vi "avitolcm.vi"() -> ()   [LabVIEW 2015]
uses:
  G_LCM.vi
panel:
  out "error out":errorcluster
  in  "Image 2":T1(plugin-control)
  in  "port":u16=7667
  in  "time-to-live":u16
  out "Image":T1(plugin-control)
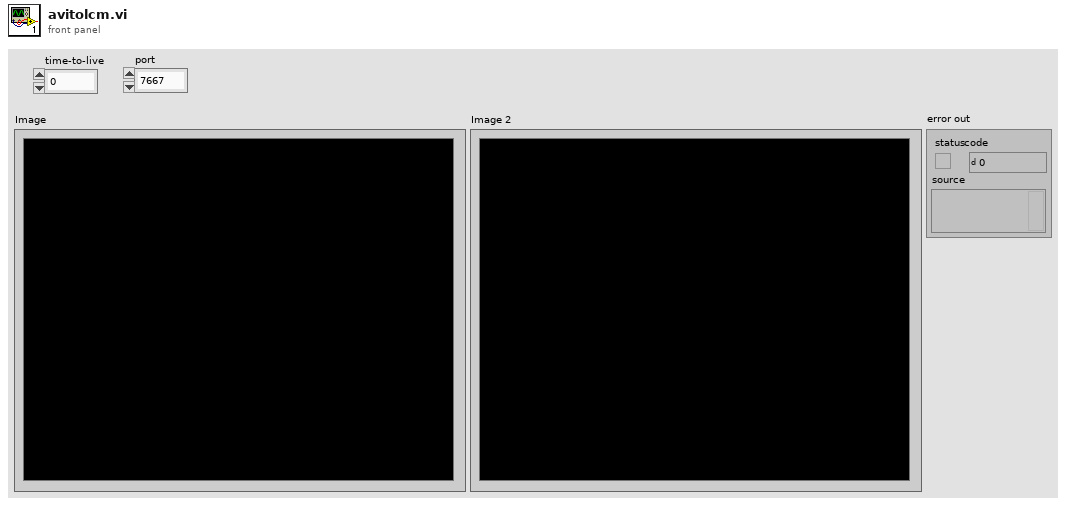
[diagram p1: front panel]
types:
  T1 = typedef "IMAQ Image.ctl" = refnum<image>
  T2 = cluster{"connection ID":refnum<k16>, "net address":u32, "port":u16}
  T3 = cluster{"hash":i64, "sys time":i64, "width":i32, "height":i32, "size":i32, "data":i32[]}
  T4 = typedef "IMAQ AVI2 Refnum.ctl" = refnum<k20>
  T5 = typedef "Image Type" = u32
  T6 = cluster{"Width":u32, "Height":u32, "Frames Per Second":u32, "Codec":string, "Has Data":bool}
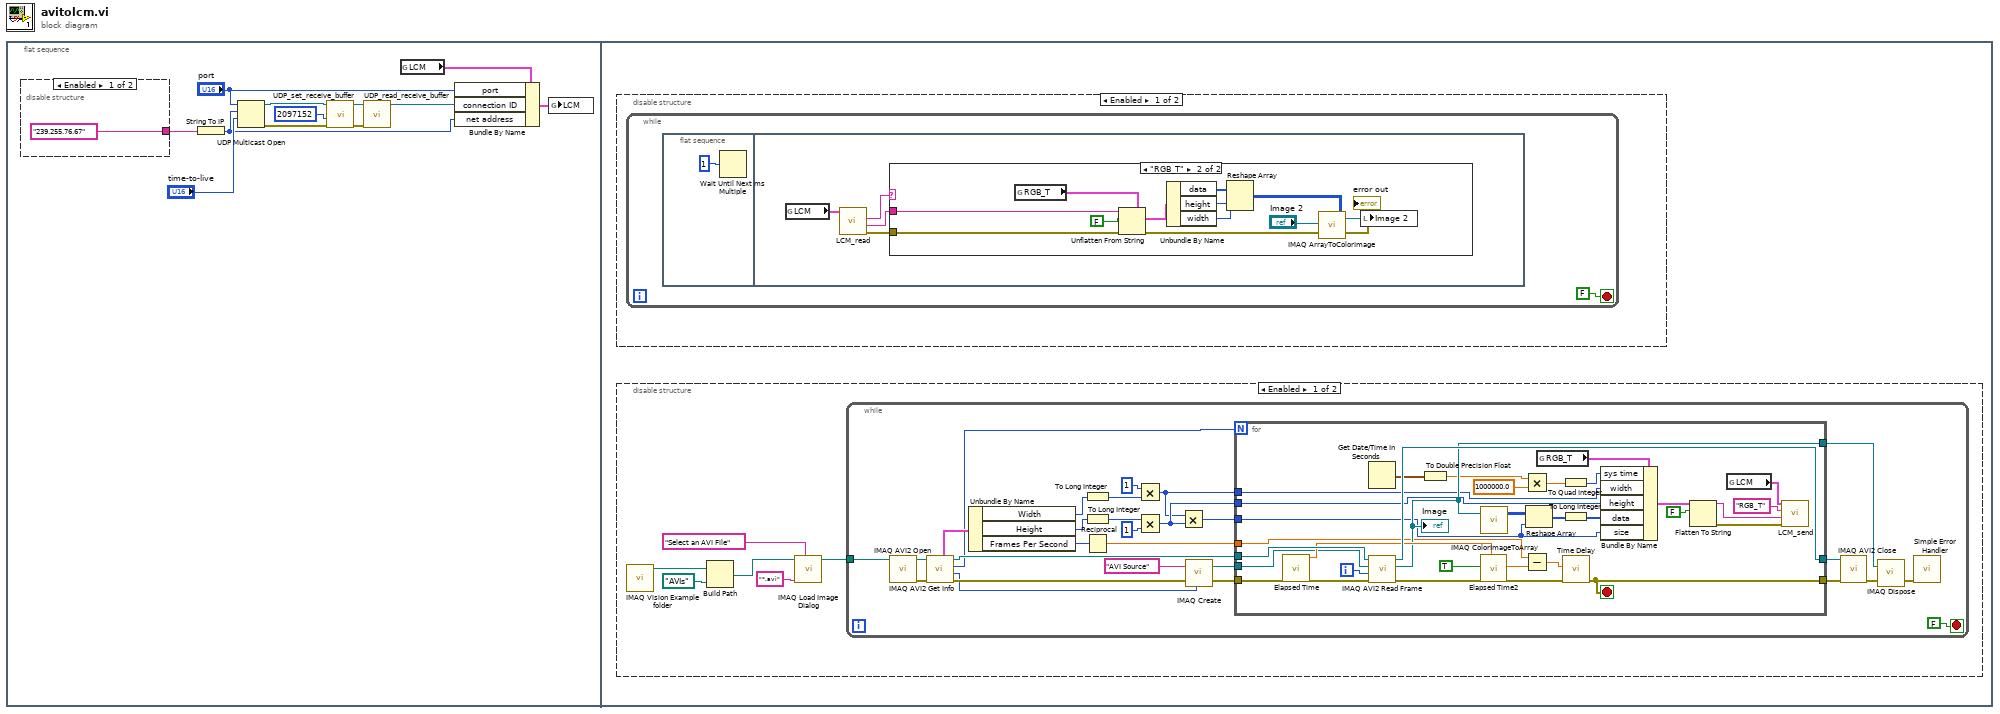
[diagram p0: block diagram]
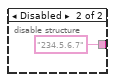
[diagram p2: hidden frame]
diagram:
  n1 = flat-sequence {
    frame #0 {
      n2 = disable-structure shown="Enabled" {
        disable-tunnel: ["239.255.76.67" ("Multicast Address") "234.5.6.7" ("Multicast Address")] -> w12
        frame Enabled {
        }
        frame Disabled {
        }
      }
      n3 = String To IP(1:w12) -> (0:w8:u32)
      n4 = UDP Multicast Open(9:"time-to-live", 10:w8, 11:"port") -> (0:w1:errorcluster, 3:w3:refnum<k16>)  [unwired: 2 in, 1 out]
      n5 = call "UDP_set_receive_buffer.vi"("error in (no error)"=w1, "Receive Buffer Size"=u32 2097152, "connection ID"=w3) -> ("error out"=w5:errorcluster, "connection ID out"=w4:refnum<k16>)  [unwired: 6 in]
      n6 = call "UDP_read_receive_buffer.vi"("error in (no error)"=w5, "connection ID"=w4) -> ("connection ID out"=w2:refnum<k16>)  [unwired: 5 in, 2 out]
      n7 = global read "G_LCM.vi" "LCM"() -> (w10:T2)
      n8 = Bundle By Name(cluster=w10, "port"="port", "connection ID"=w2, "net address"=w8) -> (w9:T2)
      n9 = global write "G_LCM.vi" "LCM"(w9) -> ()
    }
    frame #1 {
      n10 = disable-structure shown="Enabled" {
        frame Enabled {
          n11 = while {
            stop <- FALSE ("status") stop-if-true
            n12 = flat-sequence {
              frame #0 {
                n13 = Wait Until Next ms Multiple(millisecond multiple=u32 1) -> ()  [unwired: 1 out]
              }
              frame #1 {
                n14 = global read "G_LCM.vi" "LCM"() -> (w20:T2)
                n15 = call "LCM_read.vi"("LCM"=w20) -> ("error out 2"=w17:errorcluster, "data"=w18:string, "ID"=w19:string)  [unwired: 7 in, 1 out]
                n16 = case shown="\"RGB_T\"" w19 {
                  tunnel: w18 -> [_ w31]
                  tunnel: w17 -> [_ w27]
                  frame "False", Default {
                  }
                  frame "RGB_T" {
                    n17 = global read "G_LCM.vi" "RGB_T"() -> (w23:T3)
                    n18 = Unflatten From String(type=w23, binary string=w31, data includes array or string size? (T)=FALSE, error in (no error)=w27) -> (value=w32:T3, error out=w28:errorcluster)  [unwired: 1 in, 1 out]
                    n19 = Unbundle By Name(w32) -> ("data"=w22:i32[], "height"=w26:i32, "width"=w25:i32)
                    n20 = Reshape Array(w22, w26, w25) -> (w24:i32[][])
                    n21 = call "IMAQ ArrayToColorImage"("Image Pixels (U32)"=w24, "Image"="Image 2", "error in (no error)"=w28) -> ("Image Out"=w29:T1, "error out"=→"error out":errorcluster)  [unwired: 2 in]
                    n22 = local write "Image 2"(w29) -> ()
                  }
                }
              }
            }
          }
        }
        frame Disabled {
        }
      }
      n23 = disable-structure shown="Enabled" {
        frame Enabled {
          n24 = call "IMAQ Vision Example folder.vi"() -> ("Example Image Path"=w39:path)  [unwired: 11 in]
          n25 = Build Path(base path=w39, name or relative path=path "AVIs") -> (appended path=w36:path)
          n26 = call "IMAQ Load Image Dialog"("Prompt"="Select an AVI File" ("prompt"), "Pattern"="*.avi", "Start Path"=w36) -> ("Path"=w35:path)  [unwired: 6 in, 2 out]
          n27 = while {
            tunnel: w35 -> [w52]
            stop <- FALSE stop-if-true
            n28 = call "IMAQ AVI2 Open"("AVI File Path"=w52) -> ("error out"=w64:errorcluster, "AVI Refnum"=w63:T4)  [unwired: 2 in, 7 out]
            n29 = call "IMAQ AVI2 Get Info"("error in (no error)"=w64, "AVI Refnum"=w63) -> ("error out"=w60:errorcluster, "Image Type"=w55:T5, "Number of Frames"=w51:u32, "AVI Refnum (duplicate)"=w58:T4, "Frame Data"=w65:T6)  [unwired: 5 out]
            n30 = Unbundle By Name(w65) -> ("Width"=w44:u32, "Height"=w42:u32, "Frames Per Second"=w54:u32)
            n31 = To Long Integer(number=w44) -> (32bit integer=w43:i32)
            n32 = To Long Integer(number=w42) -> (32bit integer=w41:i32)
            n33 = Reciprocal(x=w54) -> (1/x=w53:dbl)
            n34 = Multiply(x=1, y=w43) -> (x*y=w46:i32)
            n35 = Multiply(x=w41, y=1) -> (x*y=w48:i32)
            n36 = Multiply(x=w46, y=w48) -> (x*y=w40:i32)
            n37 = call "IMAQ Create"("Image Name"="AVI Source", "Image Type"=w55, "error in (no error)"=w60) -> ("New Image"=w50:T1, "error out"=w59:errorcluster)  [unwired: 1 in, 1 out]
            n38 = for {
              N: w51 -> [_]
              tunnel: w50 -> [w91]
              tunnel: [w99] -> w61
              tunnel: [w68] -> w62
              tunnel: w59 -> [w98]
              tunnel: w58 -> [w100]
              tunnel: [w90] -> w56
              tunnel: w53 -> [w69]
              tunnel: w46 -> [w78]
              tunnel: w48 -> [w76]
              tunnel: w40 -> [w72]
              i -> [w92]
              stop <- w68 stop-if-true
              n39 = call "Elapsed Time"("error in (no error)"=w98) -> ("Present (s)"=w96:dbl, "error out"=w97:errorcluster)  [unwired: 11 in, 6 out]
              n40 = Get Date/Time In Seconds() -> (seconds since 1Jan1904=w88:timestamp)
              n41 = call "IMAQ AVI2 Read Frame"("error in (no error)"=w97, "Frame Number"=w92, "Image"=w91, "AVI Refnum"=w100) -> ("error out"=w94:errorcluster, "Image Out"=w90:T1, "AVI Refnum (duplicate)"=w99:T4)  [unwired: 5 out]
              "Image" <- w90
              n42 = To Double Precision Float(number=w88) -> (double precision float=w86:dbl)
              n43 = call "Elapsed Time2"("Reset"=TRUE, "error in (no error)"=w94, "Set Start Time (s)"=w96) -> ("Elapsed Time (s)"=w71:dbl, "error out"=w93:errorcluster)  [unwired: 9 in, 6 out]
              n44 = call "IMAQ ColorImageToArray"("Image"=w90) -> ("Image Pixels (U32)"=w74:u32[][])  [unwired: 3 in, 2 out]
              n45 = Multiply(x=w86, y=1000000.0) -> (x*y=w84:dbl)
              n46 = Subtract(x=w69, y=w71) -> (x-y=w70:dbl)
              n47 = Reshape Array(w74, w72) -> (w75:u32[])
              n48 = global read "G_LCM.vi" "RGB_T"() -> (w89:T3)
              n49 = To Quad Integer(1:w84) -> (0:w87:i64)
              n50 = To Long Integer(number=w75) -> (32bit integer=w73:i32[])
              n51 = call "Time Delay"("error in (no error)"=w93, "Delay Time (s)"=w70) -> ("error out"=w68:errorcluster)  [unwired: 9 in]
              n52 = Bundle By Name(cluster=w89, "sys time"=w87, "width"=w78, "height"=w76, "data"=w73, "size"=w72) -> (w83:T3)
              n53 = Flatten To String(anything=w83, prepend array or string size? (T)=FALSE) -> (data string=w77:string, error out=w82:errorcluster)  [unwired: 2 in, 1 out]
              n54 = global read "G_LCM.vi" "LCM"() -> (w81:T2)
              n55 = call "LCM_send.vi"("error in (no error)"=w82, "DATA"=w77, "ID"="RGB_T", "LCM"=w81) -> ()  [unwired: 6 in, 2 out]
            }
            n56 = call "IMAQ AVI2 Close"("error in (no error)"=w62, "AVI Refnum"=w61) -> ("error out"=w57:errorcluster)  [unwired: 9 out]
            n57 = call "IMAQ Dispose"("Image"=w56, "error in (no error)"=w57) -> ("error out"=w66:errorcluster)  [unwired: 1 in, 3 out]
            n58 = call <vilib>:"Simple Error Handler.vi"("error in (no error)"=w66) -> ()  [unwired: 1 in, 8 out]
          }
        }
        frame Disabled {
        }
      }
    }
  }
